vi "Add Buttons.vi"(8 "error in":errorcluster, 9 "Button Def JSON":path, 10 "Control Refs":T1, 11 "Button Manager in":refnum<class "Button Manager.lvclass">) -> (0 "error out":errorcluster, 3 "Button Manager out":refnum<class "Button Manager.lvclass">)   [LabVIEW 2020, in "Navigation.lvlib" / "Button Manager.lvclass"]
doc: "____\nHAMPEL SOFTWARE ENGINEERING v2.6.0 (2023-12-19 10:54)"
uses:
  Button Manager.lvclass
  Control Refs.ctl
  Button Manager.lvclass/Button Manager.ctl
  Button Def.ctl
  Top Control.ctl
  Sub Control.ctl
  <vilib>/ErrorRing/Error Ring.xnode
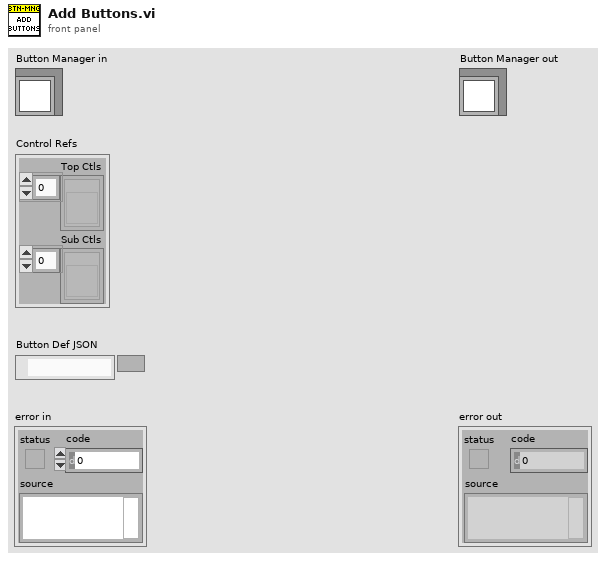
[diagram p1: front panel]
types:
  T1 = typedef "Navigation.lvlib/Button Manager.lvclass/Control Refs.ctl" = cluster{"Top Ctls":refnum<vi>[], "Sub Ctls":refnum<vi>[]}
  T2 = typedef "Navigation.lvlib/Button Manager.lvclass/Button Def.ctl" = cluster{"Top-Ctl Ref":refnum<vi>, "Sub-Ctl Ref":refnum<vi>, "Button Object":T3}
  T3 = typedef "Navigation.lvlib/Button Manager.lvclass/Top Control.ctl" = cluster{"name":string, "caption":string, "tooltip":string, "enabled_state":string, "action":string, "display_scenario":string, "sub":T4[]}
  T4 = typedef "Navigation.lvlib/Button Manager.lvclass/Sub Control.ctl" = cluster{"name":string, "tooltip":string, "enabled_state":string, "content":string[], "retain value":bool}
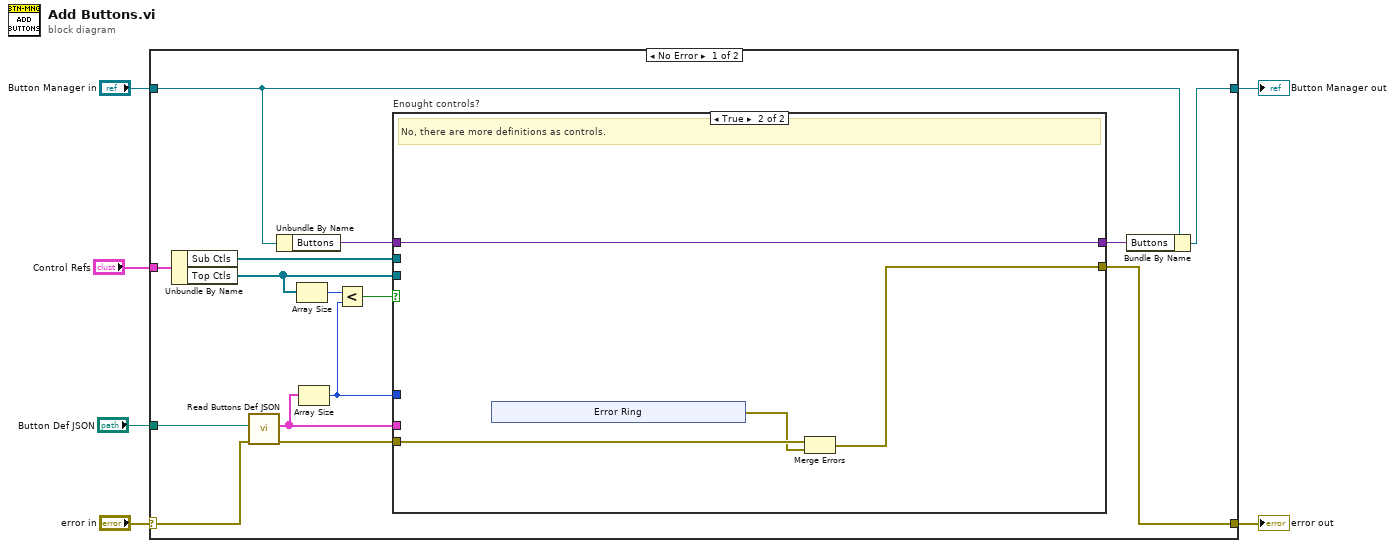
[diagram p0: block diagram]
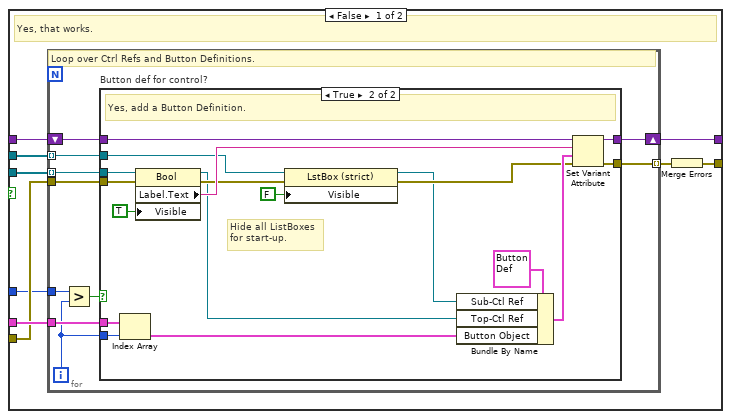
[diagram p2: hidden frame]
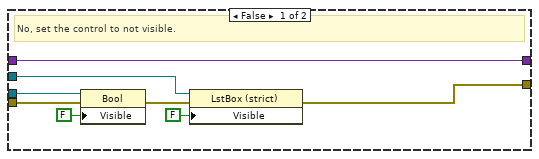
[diagram p3: hidden frame]
diagram:
  n1 = case shown="No Error" "error in" {
    selector: "error in" -> [w19 w73]
    tunnel: [w11 w73] -> w5
    tunnel: [w17 w72] -> w3
    tunnel: "Button Manager in" -> [w18 w72]
    tunnel: "Button Def JSON" -> [w20 _]
    tunnel: "Control Refs" -> [w9 _]
    frame No Error {
      n2 = Unbundle By Name(w9) -> ("Sub Ctls"=w7:refnum<vi>[], "Top Ctls"=w8:refnum<vi>[])
      n3 = call "Read Buttons Def JSON.vi"("error in"=w19, "Button Def JSON"=w20) -> ("error out"=w12:errorcluster, "Button Objects"=w15:T3[])  [unwired: 8 in]
      n4 = Unbundle By Name(w18) -> ("Buttons"=w21:variant)
      n5 = Array Size(array=w8) -> (size(s)=w14:i32)
      n6 = Array Size(array=w15) -> (size(s)=w10:i32)
      n7 = Less?(x=w14, y=w10) -> (x < y?=w13:bool)
      n8 = case "Enought controls?" shown="True" w13 {
        tunnel: w21 -> [w30 w70]
        tunnel: [w29 w70] -> w16
        tunnel: [w25 w68] -> w11
        tunnel: w8 -> [w28 _]
        tunnel: w15 -> [w27 _]
        tunnel: w12 -> [w26 w69]
        tunnel: w10 -> [w23 _]
        tunnel: w7 -> [w22 _]
        frame False {
          # "Yes, that works."
          n9 = for {
            tunnel: w27 -> [w35]
            tunnel: w28 -> [w39] mode=indexing
            tunnel: w26 -> [w38]
            shift-right: [w37] -> w29
            shift-left: w30 -> [w40]
            tunnel: [w36] -> w24 mode=indexing
            tunnel: w23 -> [w33]
            tunnel: w22 -> [w31] mode=indexing
            i -> [w34]
            # "Loop over Ctrl Refs and Button Definitions."
            n10 = Greater?(x=w33, y=w34) -> (0:w32:bool)
            n11 = case "Button def for control?" shown="True" w32 {
              tunnel: w40 -> [w48 w66]
              tunnel: w39 -> [w47 w65]
              tunnel: w38 -> [w46 w62]
              tunnel: [w48 w60] -> w37
              tunnel: [w43 w59] -> w36
              tunnel: w35 -> [_ w58]
              tunnel: w34 -> [_ w57]
              tunnel: w31 -> [w42 w53]
              frame False {
                # "No, set the control to not visible."
                n12 = property class="Bool"(reference=w47, error in=w46, "Visible"=FALSE) -> (error out=w44:errorcluster)  [unwired: 1 out]
                n13 = property class="LstBox (strict)"(reference=w42, error in=w44, "Visible"=FALSE) -> (error out=w43:errorcluster)  [unwired: 1 out]
              }
              frame True {
                # "Hide all ListBoxes\nfor start-up."
                # "Yes, add a Button Definition."
                n14 = Index Array(array=w58, index=w57) -> (element=w52:T3)
                n15 = property class="Bool"(reference=w65, error in=w62, "Visible"=TRUE) -> (reference out=w51:refnum<vi>, error out=w55:errorcluster, "Label.Text"=w64:string)
                n16 = property class="LstBox (strict)"(reference=w53, error in=w55, "Visible"=FALSE) -> (reference out=w50:refnum<vi>, error out=w54:errorcluster)
                n17 = Bundle By Name(cluster=T2 {"Top-Ctl Ref"=refnum, "Sub-Ctl Ref"=refnum, "Button Object"={"name"="", "caption"="", "tooltip"="", "enabled_state"="", "action"="", "display_scenario"="", "sub"=[]}} ("Button Def"), "Sub-Ctl Ref"=w50, "Top-Ctl Ref"=w51, "Button Object"=w52) -> (w61:T2)
                n18 = Set Variant Attribute(Variant=w66, name=w64, value=w61, error in=w54) -> (Variant out=w60:variant, error out=w59:errorcluster)  [unwired: 1 out]
              }
            }
          }
          n19 = Merge Errors(w24) -> (w25:errorcluster)
        }
        frame True {
          # "No, there are more definitions as controls."
          n20 = xnode "Error Ring"() -> ("error out"=w67:errorcluster)
          n21 = Merge Errors(w69, w67) -> (w68:errorcluster)
        }
      }
      n22 = Bundle By Name(cluster=w18, "Buttons"=w16) -> (w17:refnum<class "Button Manager.lvclass">)
    }
    frame Error {
    }
  }
  "error out" <- w5
  "Button Manager out" <- w3
